vi "count2rad.vi"(8 "error in (no error)":errorcluster, 10 "Encoder 1 Count":i32, 11 "Encoder 0 Count":i32) -> (0 "error out":errorcluster, 2 "Enc 1 angle (rad)":dbl, 3 "Enc 0 angle (rad)":dbl)   [LabVIEW 2017]
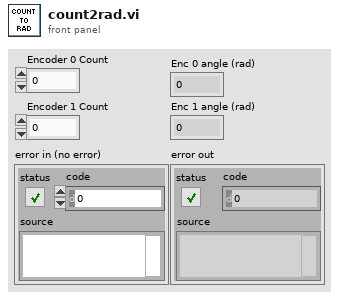
[diagram p1: front panel]
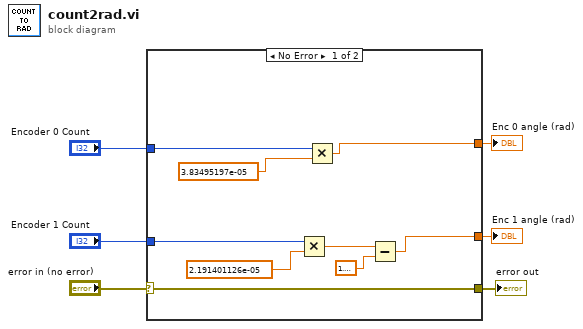
[diagram p0: block diagram]
diagram:
  n1 = case shown="No Error" "error in (no error)" {
    selector: "error in (no error)" -> [w15 w16]
    tunnel: [w15 w16] -> w5
    tunnel: "Encoder 0 Count" -> [w14 _]
    tunnel: "Encoder 1 Count" -> [w10 _]
    tunnel: [w8 _] -> w2
    tunnel: [w12 _] -> w1
    frame No Error {
      n2 = Multiply(x=w10, y=2.191401126e-05) -> (x*y=w9:dbl)
      n3 = Multiply(x=w14, y=3.83495197e-05) -> (x*y=w12:dbl)
      n4 = Subtract(x=w9, y=1.5707963267948966) -> (x-y=w8:dbl)
    }
    frame Error {
    }
  }
  "error out" <- w5
  "Enc 0 angle (rad)" <- w1
  "Enc 1 angle (rad)" <- w2
